vi "get_component_type_name.vi"(8 "error in (no error)":errorcluster, 11 "GenericSegmenter in":refnum<class "GenericSegmenter.lvclass">) -> (0 "error out":errorcluster, 2 "component type":string="Segmenter", 3 "GenericSegmenter out":refnum<class "GenericSegmenter.lvclass">)   [LabVIEW 2010, in "GenericSegmenter.lvclass"]
uses:
  GenericSegmenter.lvclass
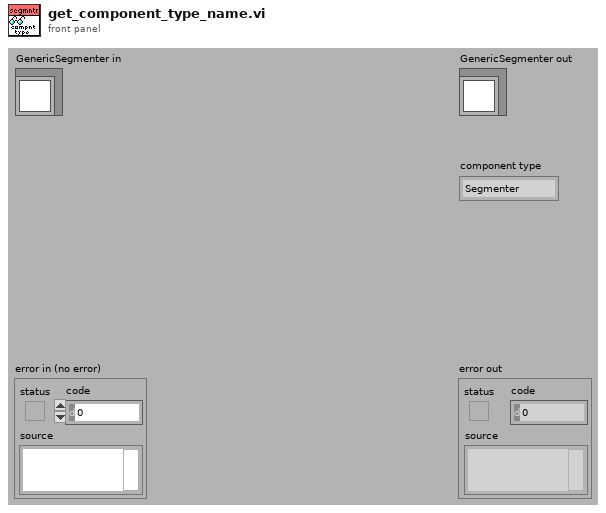
[diagram p1: front panel]
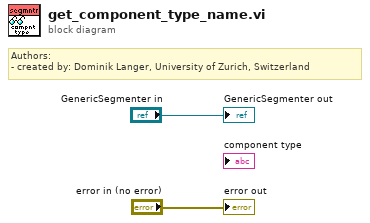
[diagram p0: block diagram]
diagram:
  # "Authors: \n- created by: Dominik Langer, University of Zurich, Switzerland"
  "error out" <- "error in (no error)"
  "GenericSegmenter out" <- "GenericSegmenter in"
